vi "PinTest RTMain.vi"() -> ()   [LabVIEW 2012]
uses:
  Type/RT Loop Events.ctl
  Type/_RW Status.ctl
  _RT Global.vi
  <vilib>/FPGAPlugInAG/sbRIO-9606/niLvFpga_Open_sbRIO-9606.vi
  <vilib>/Utility/error.llb/Error Cluster From Error Code.vi
  <vilib>/rvi/errors/niLvFpgaAdjustHostInterfaceError.vi
  <vilib>/rvi/interface/nirviOpenFPGA/nirviOpenFPGA.xnode
  FPGA Bitfiles/FPGA9606PinTest.lvbitx
  <vilib>/rvi/interface/nirviReadWriteControl/nirviReadWriteControl.xnode
  <vilib>/NI_Real-Time Target Support.lvlib
  NiFpgaLv.dll
panel:
  out "Address2":i32
  out "Data 2":u32
  out "Data":u32
  out "Address":u32
  in  "RT Version":u32=900130925
  out "FPGA Version":u32
  out "Time (s)":dbl
  out "Connected?":bool
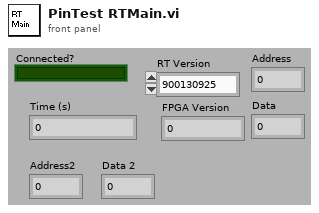
[diagram p1: front panel]
types:
  T1 = typedef "RT Loop Events.ctl" = enum16{"Initialize", "Wait for Connection", "Wait for Command", "Send Reply"}
  T2 = cluster{"Rt Loop Events":T1, "Connection ID":refnum<k5>, "Info":string, "Data Array":i32[], "error":errorcluster}
  T3 = typedef "_RW Status.ctl" = enum8{"Done", "Do Read", "Do Write", "Set Latch1", "Set Latch2", "Set Latch3", "Set Latch4", "RP ON", "EL ON", "Serial Send", "Set LC Out", "Get LC In", "Read VAC", "Table Test", "Get Interlock", "Do Read2", "Do Write2"}
  T4 = cluster{"Info":string, "Data Array":i32[], "error":errorcluster}
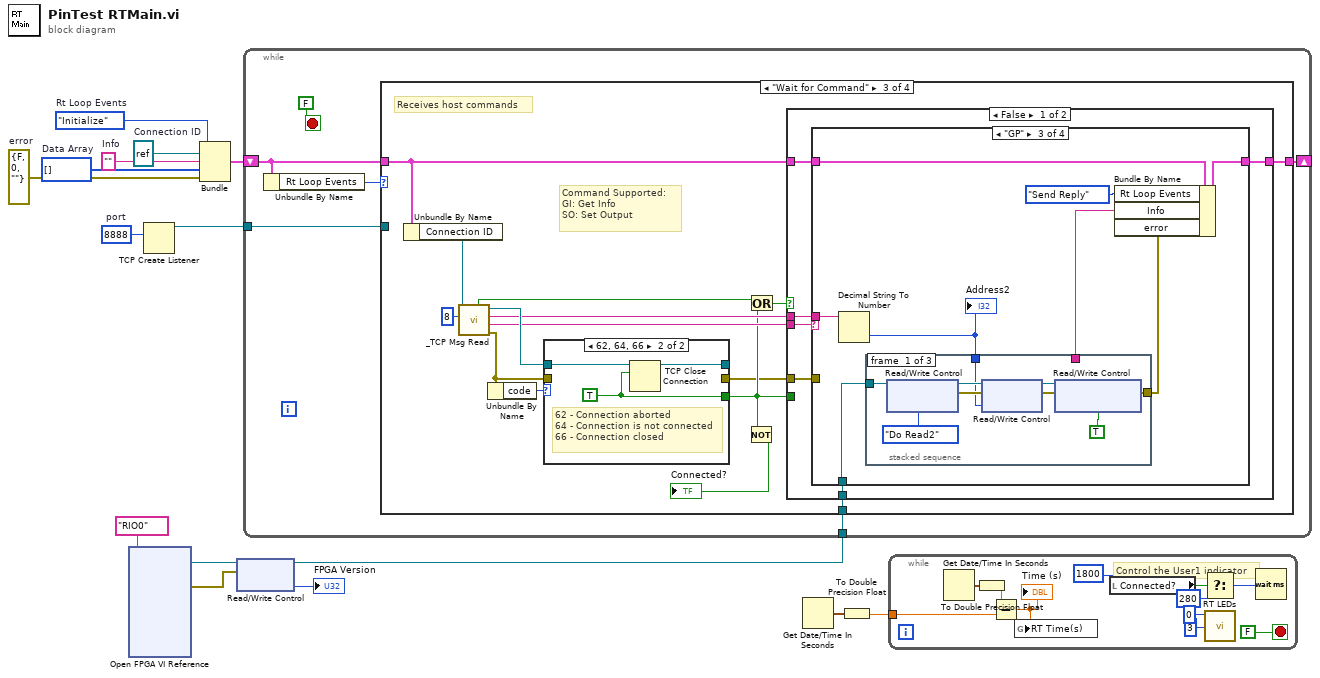
[diagram p0: block diagram]
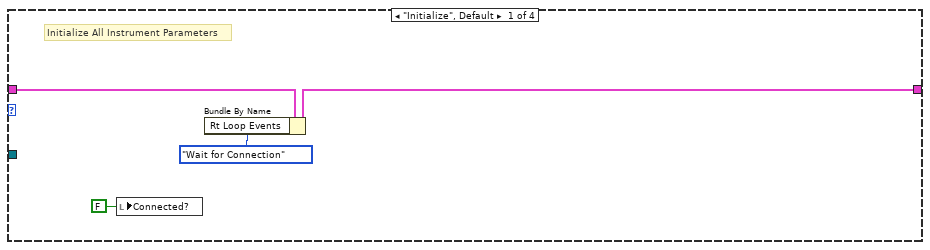
[diagram p2: hidden frame]
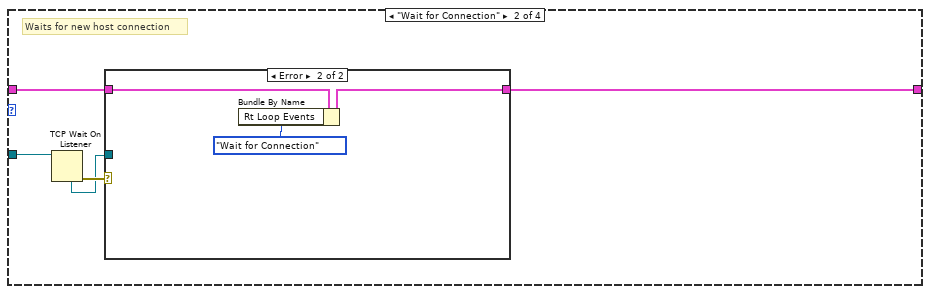
[diagram p3: hidden frame]
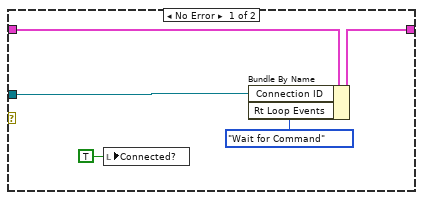
[diagram p4: hidden frame]
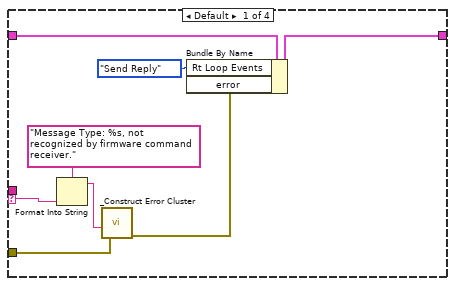
[diagram p5: hidden frame]
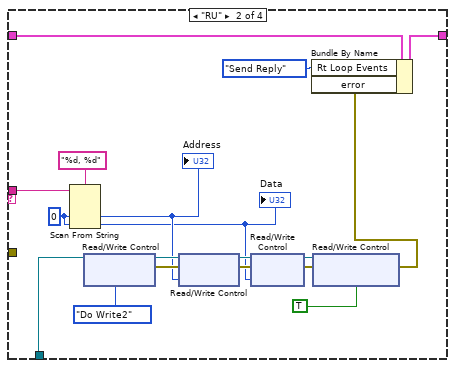
[diagram p6: hidden frame]
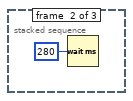
[diagram p7: hidden frame]
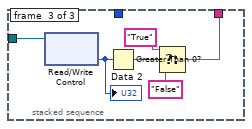
[diagram p8: hidden frame]
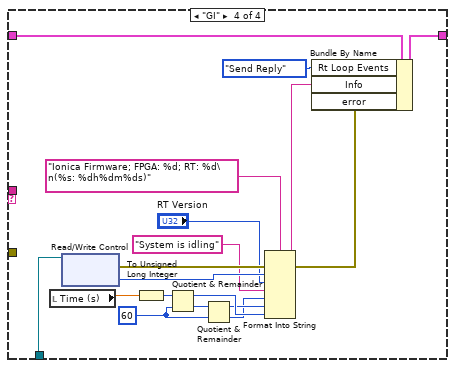
[diagram p9: hidden frame]
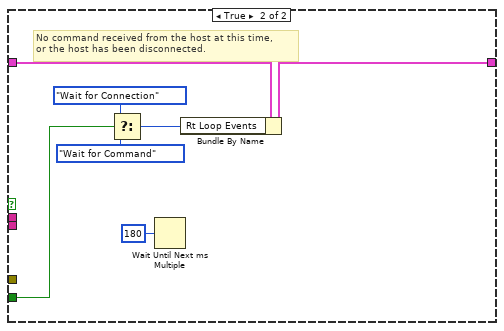
[diagram p10: hidden frame]
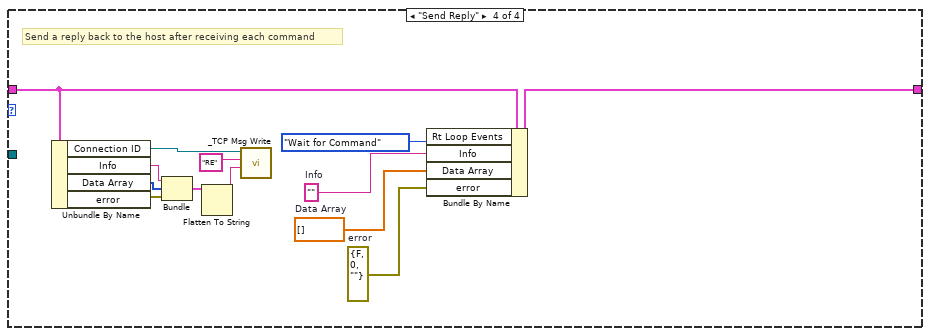
[diagram p12: hidden frame]
diagram:
  w8 = u16 8888  # port
  w10 = i32[] []  # Data Array
  w11 = ""  # Info
  w12 = errorcluster {"status"=FALSE, "code"=0, "source"=""}  # error
  w14 = refnum<k5> refnum  # Connection ID
  w15 = RT_Loop_Events."Initialize"  # Rt Loop Events
  n1 = xnode "Open FPGA VI Reference"("resource name"=tag "RIO0") -> ("FPGA VI Reference Out"=w6:refnum<k20>, "error out"=w5:errorcluster)  [unwired: 1 in]
  n2 = TCP Create Listener(10:w8) -> (3:w7:refnum<k5>)  [unwired: 4 in, 2 out]
  n3 = Bundle("Rt Loop Events"=w15, "Connection ID"=w14, "Info"=w11, "Data Array"=w10, "error"=w12) -> (w13:T2)  [unwired: 1 in]
  n4 = xnode "Read/Write Control"("FPGA VI Reference In"=w6, "error in"=w5) -> ("FPGA VI Reference Out"=w4:refnum<k20>, "Version"=→"FPGA Version":u32)  [unwired: 1 out]
  n5 = while {
    shift-right: [w18] -> _
    shift-left: w13 -> [w19]
    tunnel: w4 -> [w17]
    tunnel: w7 -> [w16]
    stop <- FALSE stop-if-true
    n6 = Unbundle By Name(w19) -> ("Rt Loop Events"=w20:T1)
    n7 = case shown="\"Wait for Command\"" w20 {
      tunnel: w19 -> [w24 w30 w49 w145]
      tunnel: [w23 w29 w48 w144] -> w18
      tunnel: w17 -> [_ _ w41 _]
      tunnel: w16 -> [_ w27 _ _]
      frame "Initialize", Default {
        # "Initialize All Instrument Parameters"
        n8 = local write "Connected?"(FALSE ("Connected?")) -> ()
        n9 = Bundle By Name(cluster=w24, "Rt Loop Events"=RT_Loop_Events."Wait for Connection") -> (w23:T2)
      }
      frame "Wait for Connection" {
        # "Waits for new host connection"
        n10 = TCP Wait On Listener(11:w27) -> (0:w28:errorcluster, 4:w26:refnum<k5>)  [unwired: 3 in, 3 out]
        n11 = case shown="Error" w28 {
          tunnel: w30 -> [w35 w38]
          tunnel: w26 -> [w32 _]
          tunnel: [w34 w36] -> w29
          frame No Error {
            n12 = local write "Connected?"(TRUE ("Connected?")) -> ()
            n13 = Bundle By Name(cluster=w35, "Connection ID"=w32, "Rt Loop Events"=RT_Loop_Events."Wait for Command") -> (w34:T2)
          }
          frame Error {
            n14 = Bundle By Name(cluster=w38, "Rt Loop Events"=RT_Loop_Events."Wait for Connection") -> (w36:T2)
          }
        }
      }
      frame "Wait for Command" {
        # "Command Supported:\nGI: Get Info\nSO: Set Output"
        # "Receives host commands"
        n15 = Unbundle By Name(w49) -> ("Connection ID"=w43:refnum<k5>)
        n16 = call "_TCP Msg Read.vi"("timeout ms (10000)"=8 ("millisecond multiple"), "connection ID"=w43) -> ("error out"=w40:errorcluster, "Message Type"=w47:string, "Data Stream"=w46:string, "connection ID out"=w52:refnum<k5>, "Timed Out?"=w51:bool)  [unwired: 3 in, 2 out]
        n17 = Unbundle By Name(w40) -> ("code"=w53:i32)
        n18 = case shown="62, 64, 66" w53 {
          tunnel: [w135 w138] -> _
          tunnel: [_ w137] -> w45
          tunnel: w52 -> [w135 w136]
          tunnel: w40 -> [w134 _]
          tunnel: [w134 _] -> w39
          frame Default {
          }
          frame 62, 64, 66 {
            w137 = TRUE ("abort (F)")
            # "62 - Connection aborted\n64 - Connection is not connected\n66 - Connection closed"
            n19 = TCP Close Connection(connection ID=w136, abort (F)=w137) -> (connection ID out=w138:refnum<k5>)  [unwired: 1 in, 1 out]
          }
        }
        n20 = Not(x=w45) -> (.not. x?=→"Connected?":bool)
        n21 = Or(x=w51, y=w45) -> (x .or. y?=w50:bool)
        n22 = case shown="False" w50 {
          tunnel: w45 -> [_ w133]
          tunnel: w49 -> [w58 w132]
          tunnel: [w57 w131] -> w48
          tunnel: w47 -> [w55 _]
          tunnel: w46 -> [w59 _]
          tunnel: w41 -> [w56 _]
          tunnel: w39 -> [w54 _]
          frame False {
            n23 = case shown="\"GP\"" w55 {
              selector: w55 -> [w67 _ _ _]
              tunnel: w59 -> [_ w82 w89 _]
              tunnel: w58 -> [w63 w84 w92 w125]
              tunnel: [w62 w83 w91 w124] -> w57
              tunnel: w56 -> [_ w73 w90 w123]
              tunnel: w54 -> [w60 _ _ _]
              frame Default {
                n24 = Format Into String(format string="Message Type: %s, not recognized by firmware command receiver.", w67) -> (resulting string=w65:string)  [unwired: 2 in, 1 out]
                n25 = call "_Construct Error Cluster.vi"("error in"=w60, "reason"=w65) -> ("error out"=w61:errorcluster)  [unwired: 5 in]
                n26 = Bundle By Name(cluster=w63, "Rt Loop Events"=RT_Loop_Events."Send Reply", "error"=w61) -> (w62:T2)
              }
              frame "RU" {
                w80 = u32 0 ("default value 1")
                n27 = Scan From String(format string="%d, %d", input string=w82, default 1=w80, default 2=w80) -> (output 1=w71:u32, output 2=w70:u32)  [unwired: 2 in, 3 out]
                "Address" <- w71
                "Data" <- w70
                n28 = xnode "Read/Write Control"("FPGA VI Reference In"=w73, "RW Status"=_RW_Status."Do Write2") -> ("FPGA VI Reference Out"=w79:refnum<k20>, "error out"=w78:errorcluster)  [unwired: 1 in]
                n29 = xnode "Read/Write Control"("FPGA VI Reference In"=w79, "error in"=w78, "Address"=w71) -> ("FPGA VI Reference Out"=w77:refnum<k20>, "error out"=w76:errorcluster)
                n30 = xnode "Read/Write Control"("FPGA VI Reference In"=w77, "error in"=w76, "Data"=w70) -> ("FPGA VI Reference Out"=w75:refnum<k20>, "error out"=w74:errorcluster)
                n31 = xnode "Read/Write Control"("FPGA VI Reference In"=w75, "error in"=w74, "Read/Write 2"=TRUE) -> ("error out"=w68:errorcluster)  [unwired: 1 out]
                n32 = Bundle By Name(cluster=w84, "Rt Loop Events"=RT_Loop_Events."Send Reply", "error"=w68) -> (w83:T2)
              }
              frame "GP" {
                n33 = Decimal String To Number(string=w89) -> (number=w88:i32)  [unwired: 3 out]
                "Address2" <- w88
                n34 = stacked-sequence {
                  tunnel: w90 -> [w100 _ w109]
                  tunnel: [w97 _ _] -> w87
                  tunnel: w88 -> [w96 _ _]
                  tunnel: [_ _ w104] -> w86
                  frame #0 {
                    n35 = xnode "Read/Write Control"("FPGA VI Reference In"=w100, "RW Status"=_RW_Status."Do Read2") -> ("FPGA VI Reference Out"=w102:refnum<k20>, "error out"=w101:errorcluster)  [unwired: 1 in]
                    n36 = xnode "Read/Write Control"("FPGA VI Reference In"=w102, "error in"=w101, "Address"=w96) -> ("FPGA VI Reference Out"=w95:refnum<k20>, "error out"=w94:errorcluster)
                    n37 = xnode "Read/Write Control"("FPGA VI Reference In"=w95, "error in"=w94, "Read/Write 2"=TRUE) -> ("error out"=w97:errorcluster)  [unwired: 1 out]
                  }
                  frame #1 {
                    n38 = Wait (ms)(milliseconds to wait=u32 280) -> ()  [unwired: 1 out]
                  }
                  frame #2 {
                    n39 = xnode "Read/Write Control"("FPGA VI Reference In"=w109) -> ("Data"=w108:u32)  [unwired: 1 in, 2 out]
                    "Data 2" <- w108
                    n40 = Greater Than 0?(x=w108) -> (x > 0?=w107:bool)
                    n41 = Select(t="True", s=w107, f="False") -> (s? t:f=w104:string)
                  }
                }
                n42 = Bundle By Name(cluster=w92, "Rt Loop Events"=RT_Loop_Events."Send Reply", "Info"=w86, "error"=w87) -> (w91:T2)
              }
              frame "GI" {
                w111 = u32 60 ("Time (s)")
                n43 = local read "Time (s)"() -> (w112:dbl)
                n44 = xnode "Read/Write Control"("FPGA VI Reference In"=w123) -> ("error out"=w122:errorcluster, "Version"=w115:u32)  [unwired: 1 in, 1 out]
                n45 = To Unsigned Long Integer(number=w112) -> (unsigned 32bit integer=w121:u32)
                n46 = Quotient & Remainder(x=w121, y=w111) -> (x-y*floor(x/y)=w119:u32, floor(x/y)=w120:u32)
                n47 = Quotient & Remainder(x=w120, y=w111) -> (x-y*floor(x/y)=w118:u32, floor(x/y)=w117:u32)
                n48 = Format Into String(format string="Ionica Firmware; FPGA: %d; RT: %d\n(%s: %dh%dm%ds)", w115, "RT Version", "System is idling", w117, w118, w119) -> (resulting string=w110:string)  [unwired: 2 in, 1 out]
                n49 = Bundle By Name(cluster=w125, "Rt Loop Events"=RT_Loop_Events."Send Reply", "Info"=w110, "error"=w122) -> (w124:T2)
              }
            }
          }
          frame True {
            # "No command received from the host at this time,\nor the host has been disconnected."
            n50 = Select(t=RT_Loop_Events."Wait for Connection" ("Rt Loop Events"), s=w133, f=RT_Loop_Events."Wait for Command") -> (s? t:f=w128:T1)
            n51 = Wait Until Next ms Multiple(millisecond multiple=u32 180 ("milliseconds to wait")) -> ()  [unwired: 1 out]
            n52 = Bundle By Name(cluster=w132, "Rt Loop Events"=w128) -> (w131:T2)
          }
        }
      }
      frame "Send Reply" {
        w142 = sgl[] []  # Data Array
        w140 = errorcluster {"status"=FALSE, "code"=0, "source"=""}  # error
        w143 = ""  # Info
        # "Send a reply back to the host after receiving each command"
        n53 = Unbundle By Name(w145) -> ("Connection ID"=w147:refnum<k5>, "Info"=w148:string, "Data Array"=w151:i32[], "error"=w141:errorcluster)
        n54 = Bundle("Info"=w148, "Data Array"=w151, "error"=w141) -> (w139:T4)  [unwired: 1 in]
        n55 = Flatten To String(anything=w139) -> (data string=w149:string)  [unwired: 3 in, 2 out]
        n56 = call "_TCP Msg Write.vi"("Data Stream"=w149, "Message Type"="RE" ("Name"), "connection ID"=w147) -> ()  [unwired: 5 in, 4 out]
        n57 = Bundle By Name(cluster=w145, "Rt Loop Events"=RT_Loop_Events."Wait for Command", "Info"=w143, "Data Array"=w142, "error"=w140) -> (w144:T2)
      }
    }
  }
  n58 = Get Date/Time In Seconds() -> (seconds since 1Jan1904=w1:timestamp)
  n59 = To Double Precision Float(number=w1) -> (double precision float=w2:dbl)
  n60 = while {
    tunnel: w2 -> [w153]
    stop <- FALSE stop-if-true
    # "Control the User1 indicator"
    n61 = Get Date/Time In Seconds() -> (seconds since 1Jan1904=w154:timestamp)
    n62 = To Double Precision Float(number=w154) -> (double precision float=w155:dbl)
    n63 = Subtract(x=w155, y=w153) -> (x-y=w152:dbl)
    "Time (s)" <- w152
    n64 = global write "_RT Global.vi" "RT Time(s)"(w152) -> ()
    n65 = local read "Connected?"() -> (w160:bool)
    n66 = Select(t=u32 1800 ("milliseconds to wait"), s=w160, f=u32 280 ("milliseconds to wait")) -> (s? t:f=w162:u32)
    n67 = call <vilib>:"RT LEDs.vi"("State"=3, "LED Num"=0) -> ()  [unwired: 4 in, 2 out]
    n68 = Wait (ms)(milliseconds to wait=w162) -> ()  [unwired: 1 out]
  }
